vi "Motor_Plus_Impedance_controller_thursday2.vi"() -> ()   [LabVIEW 2016]
uses:
  <vilib>/Platform/TimedLoop/XDataNode/timing_clust.ctl
  <vilib>/Platform/TimedLoop/XDataNode/nitl_modes.ctl
  <vilib>/Platform/TimedLoop/XDataNode/wakeup.ctl
  <vilib>/Platform/TimedLoop/XDataNode/loadnilvce.vi
  <vilib>/Motion/Express/_s/nimc.ax.power.power.axis.vi
  <vilib>/Motion/Express/_s/nimc.fb.read.readExecutionData.axis.vi
  <vilib>/Motion/Express/_s/nimc.fb.straightLineMove.startStraightLineMove.axis.modeVelocity.0.vi
  <vilib>/Motion/Express/_s/nimc.fb.resetPosition.resetPosition.axis.vi
  <vilib>/Motion/Express/_s/nimc.fb.stopMove.stop.axis.modeDecelerate.vi
  <vilib>/Motion/Express/_s/nimc.ex.power.power.axis.vi
  <vilib>/platform/TimedLoop/XDataNode/XDataNode.xnode
  <vilib>/Motion/BlockNode/FB.NIMotion.xnode
  <vilib>/Platform/TimedLoop/XDataNode/XDNodeRunTimeDep.lvlib
panel:
  in  "Gravity":dbl format="%#_13g"
  out "Numeric 3":dbl format="%#_13g"
  out "Numeric 2":dbl format="%#_13g"
  in  "Position 2":dbl=0.25 format="%#_13g"
  out "Adjusted Motor Velocity":dbl format="%.3f"
  out "Adjusted Velocity":dbl(knob) scale=0.0..3.0
  in  "Reset Position":bool
  in  "Position":dbl=0.25 format="%#_13g"
  in  "Speed":dbl=0.25 format="%#_12g"
  out "Torque":dbl(knob) scale=-5.0..5.0
  out "Position":dbl(knob) scale=0.0..1.0
  out "Velocity":dbl(knob) scale=0.0..5.0
  out "Load Cell":dbl(knob) scale=0.0..10.0
  in  "Move to Position?":bool
  out "Load cell, V":dbl format="%.3f"
  out "motor torque, Nm":dbl format="%.3f"
  out "motor velocity, rev/s":dbl format="%.3f"
  out "motor position, rev":dbl format="%.3f"
  in  "STOP VI":bool
  in  "Enable Axis \nControl":bool
  in  "Enable Motor \nDrive":bool
  in  "EMERGENCY MOTOR STOP":bool
  # "Raw Data from System"
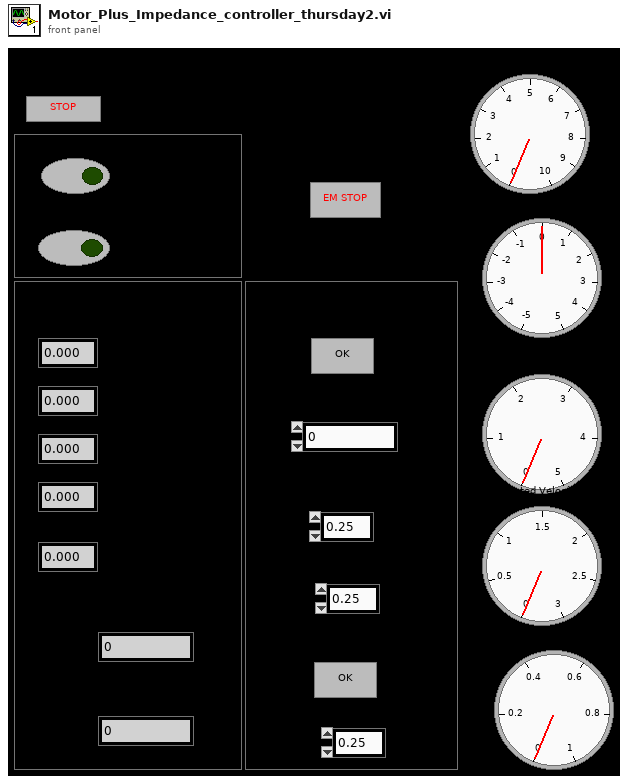
[diagram p1: front panel]
types:
  T1 = typedef "XDNodeRunTimeDep.lvlib/timing_clust.ctl" = cluster{"Expected End [f-1]":u64, "Actual End [f-1]":u64, "Finished Late? [f-1]":bool, "Expected End [i-1]":u64, "Actual End [i-1]":u64, "Finished Late? [i-1]":bool, "Expected Start [i]":u64, "Actual Start [i]":u64, "Expected Start [f]":u64, "Actual Start [f]":u64, "Source Name":string, "Structure Name":string, "Period":i64, "Deadline":i64, "Offset":i64, "Start":i64, "Priority":i32, "Timeout":i32, "Mode":T2, "Wakeup Reason":T3, "Error":errorcluster, "Source Type":string, "Secondary Source Type":string, "Global End Time":u64, "Global Start Time":u64, "Frame Duration":u64, "Iteration Duration":u64, "Assigned CPU":i32, "I/O Scan Engine Mode":u32}
  T2 = typedef "XDNodeRunTimeDep.lvlib/nitl_modes.ctl" = enum32{"No Change", "Process missed periods, maintain original phase", "Discard missed periods, maintain original phase", "Process missed periods, ignore original phase", "Discard missed periods, ignore original phase"}
  T3 = typedef "XDNodeRunTimeDep.lvlib/wakeup.ctl" = enum32{"Normal", "Aborted", "Asynchronous wakeup", "Timing source error", "Timed loop error", "Timeout"}
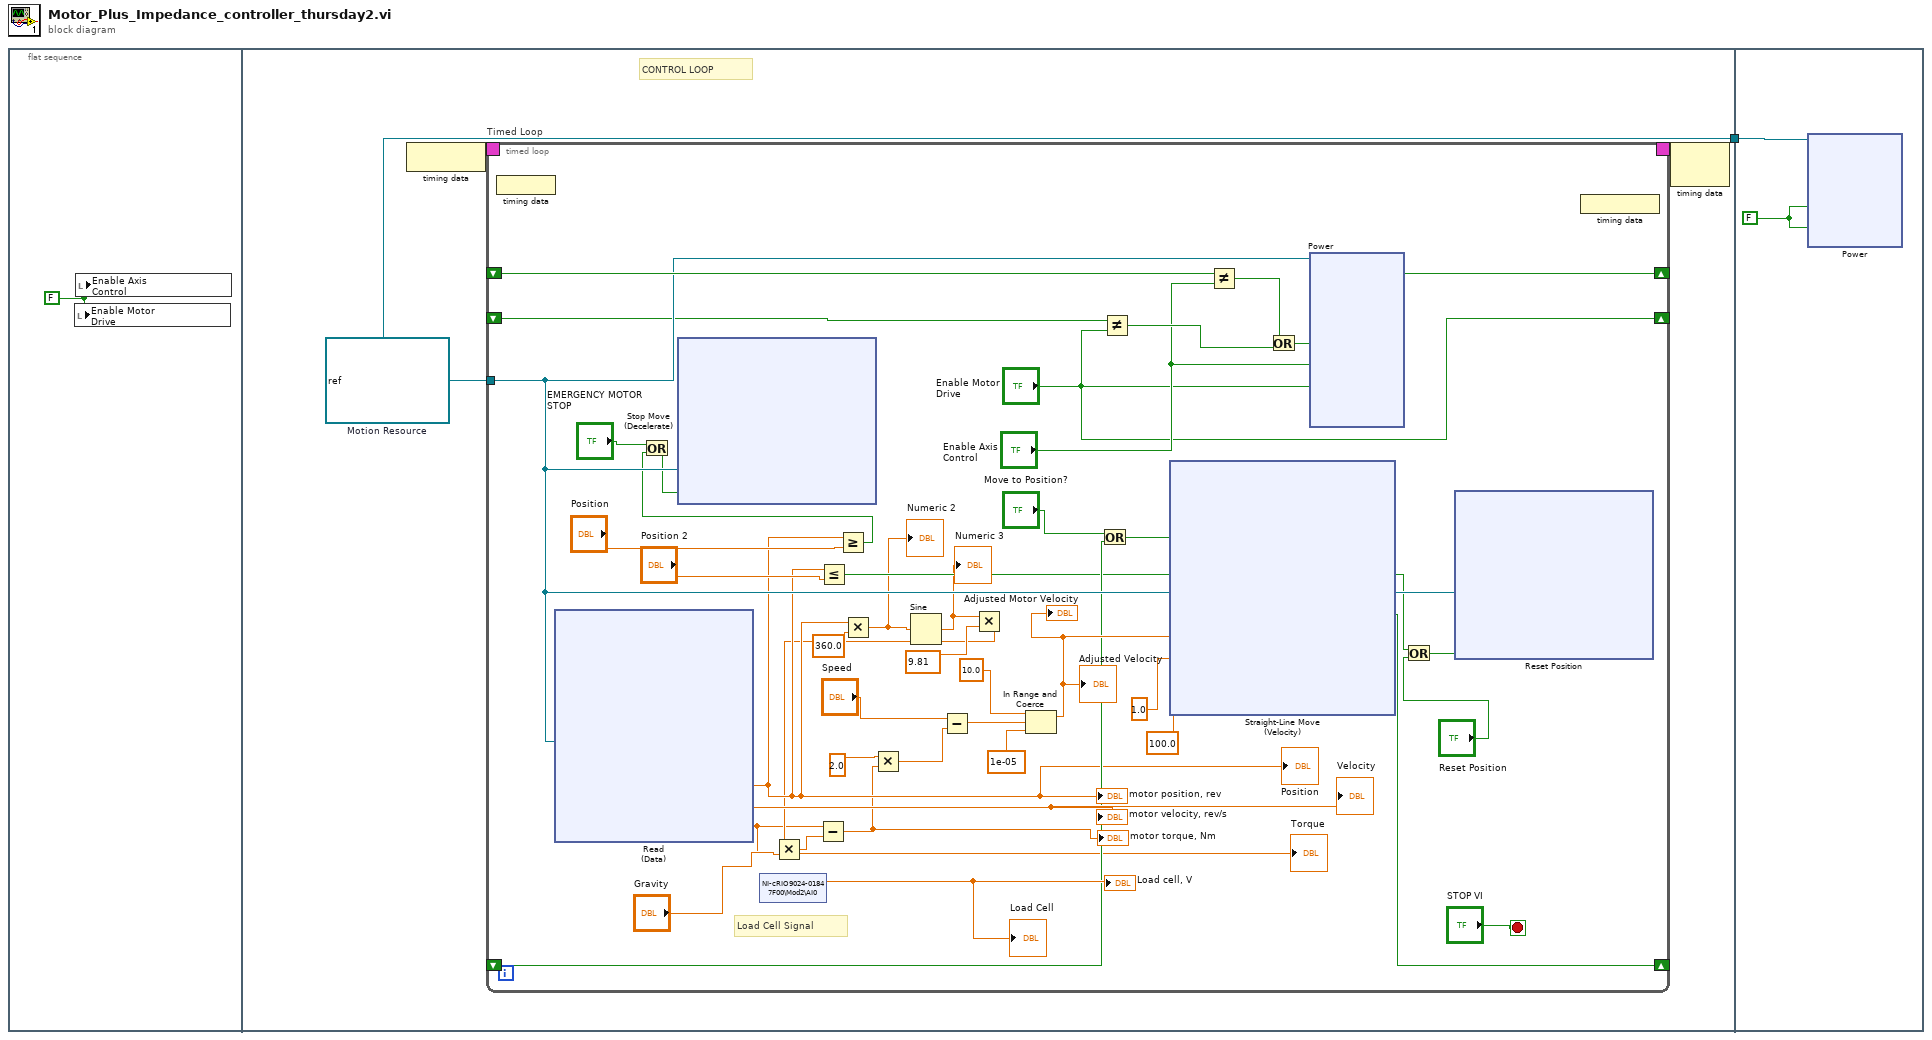
[diagram p0: block diagram]
diagram:
  n1 = flat-sequence {
    tunnel: [w5] -> w1
    tunnel: w1 -> [w126]
    frame #0 {
      w2 = FALSE
      n2 = local write "Enable Motor \nDrive"(w2) -> ()
      n3 = local write "Enable Axis \nControl"(w2) -> ()
    }
    frame #1 {
      w5 = refnum<k21> "nism://NI-cRIO9024-01847F00/Axis 1"  # Motion Resource
      # "CONTROL LOOP"
      n4 = node-c288() -> (w4:T1)
      n5 = timed-loop "Timed Loop" {
        tunnel: w5 -> [w40]
        timing: w4 -> [_]
        timing-out: [_] -> w3
        shift-right: ["Enable Axis \nControl"] -> _
        shift-left: _ -> [w47]
        shift-right: ["Enable Motor \nDrive"] -> _
        shift-left: _ -> [w22]
        shift-right: [w21] -> _
        shift-left: _ -> [w20]
        stop <- "STOP VI" stop-if-true
        # "Load Cell Signal"
        n6 = node-c288() -> ()  [unwired: 1 in]
        n7 = xnode "Read\n(Data)"("resource"=w40) -> ("position"=w15:dbl, "torque"=w6:dbl, "velocity"=→"motor velocity, rev/s" →"Velocity":dbl)  [unwired: 1 in, 3 out]
        "motor position, rev" <- w15
        "Position" <- w15
        "Torque" <- w6
        n8 = shared-variable "NI-cRIO9024-01847F00\\Mod2\\AI0"() -> (→"Load cell, V" →"Load Cell":dbl)  [unwired: 1 in, 1 out]
        n9 = Less Or Equal?(x=w15, y="Position 2") -> (x <= y?=w16:bool)
        n10 = Greater Or Equal?(x=w15, y="Position") -> (x >= y?=w17:bool)
        n11 = Or(x="EMERGENCY MOTOR STOP", y=w17) -> (x .or. y?=w30:bool)
        n12 = xnode "Stop Move\n(Decelerate)"("resource"=w40, "execute"=w30) -> ()  [unwired: 1 in, 3 out]
        n13 = Multiply(x=w15, y=360.0) -> (x*y=w13:dbl)
        "Numeric 2" <- w13
        n14 = Sine(x=w13) -> (sin(x)=w11:dbl)
        "Numeric 3" <- w11
        n15 = Multiply(x=w11, y=9.81) -> (x*y=w10:dbl)
        n16 = Multiply(x=w10, y="Gravity") -> (x*y=w8:dbl)
        n17 = Subtract(x=w6, y=w8) -> (x-y=w7:dbl)
        "motor torque, Nm" <- w7
        n18 = Multiply(x=2.0 ("Speed 2"), y=w7) -> (x*y=w24:dbl)
        n19 = Subtract(x="Speed", y=w24) -> (x-y=w27:dbl)
        n20 = In Range and Coerce(upper limit=10.0, x=w27, lower limit=1e-05) -> (coerced(x)=w32:dbl)  [unwired: 1 out]
        "Adjusted Velocity" <- w32
        "Adjusted Motor Velocity" <- w32
        n21 = Or(x="Move to Position?", y=w20) -> (x .or. y?=w18:bool)
        n22 = Not Equal?(x=w22, y="Enable Motor \nDrive") -> (x != y?=w45:bool)
        n23 = xnode "Straight-Line Move\n(Velocity)"("resource"=w40, "execute"=w18, "velocity"=w32, "acceleration"=1.0, "deceleration"=100.0) -> ("resource out"=w36:refnum<k21>, "done"=w21:bool)  [unwired: 1 in, 1 out]
        n24 = Not Equal?(x=w47, y="Enable Axis \nControl") -> (x != y?=w46:bool)
        n25 = Or(x=w46, y=w45) -> (x .or. y?=w44:bool)
        n26 = xnode ("Power")("execute"=w44, "enable axis"="Enable Axis \nControl", "enable drive"="Enable Motor \nDrive", "resource"=w40) -> ()  [unwired: 1 in, 6 out]
        n27 = Or(x=w16, y="Reset Position") -> (x .or. y?=w35:bool)
        n28 = xnode "Reset Position"("resource"=w36, "execute"=w35) -> ()  [unwired: 2 in, 3 out]
        n29 = node-c288() -> ()  [unwired: 1 out]
      }
      n30 = node-c288(w3) -> ()  [unwired: 1 out]
    }
    frame #2 {
      w127 = FALSE
      n31 = xnode ("Power")("enable axis"=w127, "enable drive"=w127, "resource"=w126) -> ()  [unwired: 1 in, 2 out]
    }
  }
